vi "tdms path to plotter png path.vi"(8 "error in":errorcluster, 10 "plotter name":string, 11 "TDMS Path":path) -> (0 "error out":errorcluster, 2 "binned plotter png save path":path, 3 "plotter png save path":path)   [LabVIEW 2013]
panel:
  out "filename without extension":string
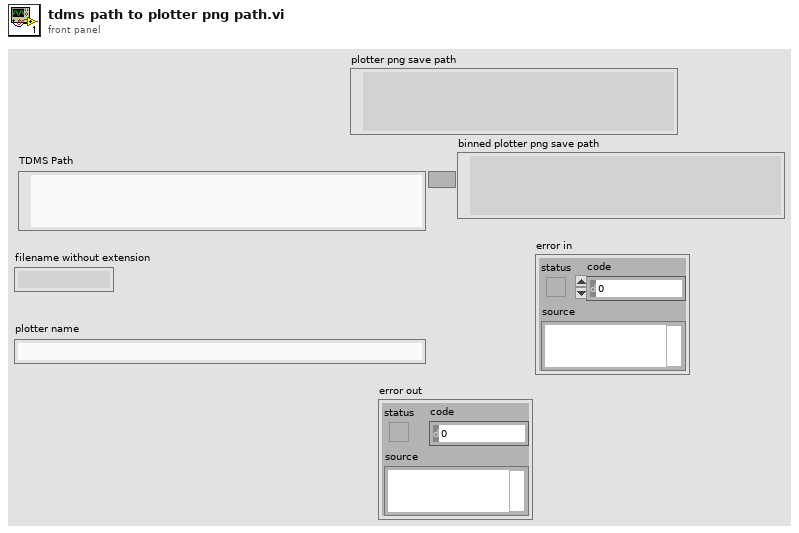
[diagram p1: front panel]
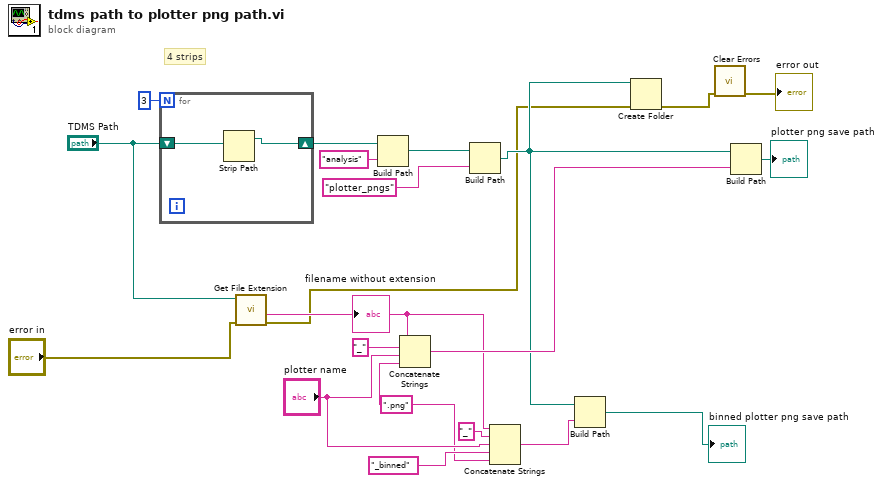
[diagram p0: block diagram]
diagram:
  w7 = ".png" ("string")
  # "4 strips"
  n1 = for {
    N: 3 -> [_]
    shift-right: [w22] -> w20
    shift-left: "TDMS Path" -> [w23]
    n2 = Strip Path(path=w23) -> (stripped path=w22:path)  [unwired: 1 out]
  }
  n3 = call <vilib>:"Get File Extension.vi"("error in (no error)"="error in", "file"="TDMS Path") -> ("error out"=w3:errorcluster, "filename without extension"=w11:string)  [unwired: 6 in, 2 out]
  "filename without extension" <- w11
  n4 = Build Path(base path=w20, name or relative path="analysis") -> (appended path=w16:path)
  n5 = Concatenate Strings(w11, "_" ("string"), "plotter name", w7) -> (w14:string)
  n6 = Build Path(base path=w16, name or relative path="plotter_pngs") -> (appended path=w5:path)
  n7 = Concatenate Strings(w11, "_" ("string"), "plotter name", "_binned" ("string"), w7) -> (w6:string)
  n8 = Build Path(base path=w5, name or relative path=w6) -> (appended path=→"binned plotter png save path":path)
  n9 = Create Folder(path (use dialog)=w5, error in=w3) -> (error out=w2:errorcluster)  [unwired: 1 in, 2 out]
  n10 = call <vilib>:"Clear Errors.vi"("error in (no error)"=w2) -> ("error out"=→"error out":errorcluster)  [unwired: 6 in]
  n11 = Build Path(base path=w5, name or relative path=w14) -> (appended path=→"plotter png save path":path)
